vi "path_selector.vi"(7 "Selector":enum16{"Direct", "Invert"}(ring), 9 "GB test time":dbl min=0.0 format="%.2f", 10 "Hi-Pot test time":dbl min=0.0 format="%.2f") -> (1 "T2":dbl min=0.0 format="%.2f", 2 "T1":dbl min=0.0 format="%.2f")   [LabVIEW 2015]
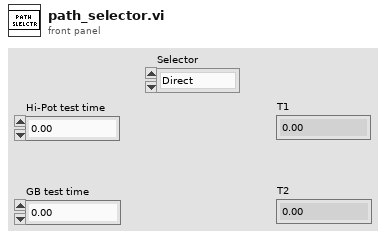
[diagram p1: front panel]
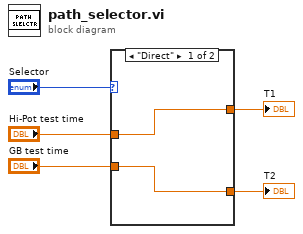
[diagram p0: block diagram]
diagram:
  n1 = case shown="\"Direct\"" "Selector" {
    tunnel: "Hi-Pot test time" -> [w7 w9]
    tunnel: "GB test time" -> [w6 w8]
    tunnel: [w6 w9] -> w2
    tunnel: [w7 w8] -> w1
    frame "Direct" {
    }
    frame "Invert" {
    }
  }
  "T2" <- w2
  "T1" <- w1
